vi "RT PID-DataLog - LED.vi"() -> ()   [LabVIEW 2017]
doc: "This example demonstrates how to simulate a general PID controller with alarms."
uses:
  <vilib>/Platform/TimedLoop/XDataNode/timing_clust.ctl
  <vilib>/Platform/TimedLoop/XDataNode/nitl_modes.ctl
  <vilib>/Platform/TimedLoop/XDataNode/wakeup.ctl
  <vilib>/addons/control/pid/pid.llb/PID (DBL).vi
  LogData.vi
  <vilib>/Utility/file.llb/Write Delimited Spreadsheet (DBL).vi
  <vilib>/Utility/file.llb/Write Delimited Spreadsheet (string).vi
  <vilib>/platform/TimedLoop/XDataNode/XDataNode.xnode
  <vilib>/addons/control/pid/NI_PID_pid.lvlib
  <vilib>/Platform/TimedLoop/XDataNode/XDNodeRunTimeDep.lvlib
panel:
  out "SP: Display":dbl(slide)=54.966887417218544 min=0.0 max=0.0 scale=0.0..100.0
  in  "Data Log Rate (ms)":u32=5000
  out "DataLog Loop stop":bool
  out "Data Log Loop ms":u32=5001
  out "PID Loop ms":u32=20
  in  "stop":bool
  out "Low Limit":bool
  out "High Limit":bool
  out "MV:":dbl(slide)=100.0 scale=-100.0..100.0
  out "PV:":dbl(slide)=33.01408837398299 scale=0.0..100.0
  in  "PID gains":T1={"proportional gain (Kc)"=20.0, "integral time (Ti, min)"=0.008, "derivative time (Td, min)"=0.001} {"derivative time (Td, min)" format="%.3f"; "integral time (Ti, min)" format="%.3f"; "proportional gain (Kc)" format="%.3f"}
  # "Overview: This example demonstrates how to simulate a general PID controller with alarms.\nInstructions:\n1. Run the VI and observe the Process Variable (PV) following the Setpoint (SP) value.\n2. Move the setpoint above or below the High Limit (HL) or Low Limit (LL). Verify the controls flashing when limits are reached.\n3. Change the Alarm limits to a value above or below if you are changing HL or LL, respectively and verify that the controller stop flashing.\n3. Click Stop to stop the VI."
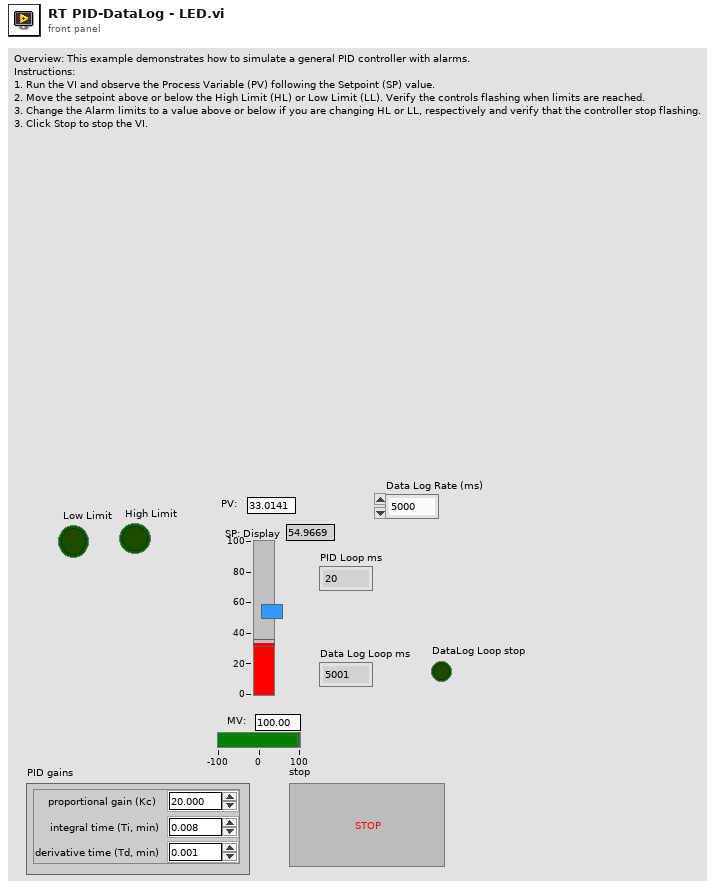
[diagram p1: front panel]
types:
  T1 = cluster{"proportional gain (Kc)":dbl, "integral time (Ti, min)":dbl, "derivative time (Td, min)":dbl}
  T2 = typedef "XDNodeRunTimeDep.lvlib/timing_clust.ctl" = cluster{"Expected End [f-1]":u64, "Actual End [f-1]":u64, "Finished Late? [f-1]":bool, "Expected End [i-1]":u64, "Actual End [i-1]":u64, "Finished Late? [i-1]":bool, "Expected Start [i]":u64, "Actual Start [i]":u64, "Expected Start [f]":u64, "Actual Start [f]":u64, "Source Name":string, "Structure Name":string, "Period":i64, "Deadline":i64, "Offset":i64, "Start":i64, "Priority":i32, "Timeout":i32, "Mode":T3, "Wakeup Reason":T4, "Error":errorcluster, "Source Type":string, "Secondary Source Type":string, "Global End Time":u64, "Global Start Time":u64, "Frame Duration":u64, "Iteration Duration":u64, "Assigned CPU":i32, "I/O Scan Engine Mode":u32}
  T3 = typedef "XDNodeRunTimeDep.lvlib/nitl_modes.ctl" = enum32{"No Change", "Process missed periods, maintain original phase", "Discard missed periods, maintain original phase", "Process missed periods, ignore original phase", "Discard missed periods, ignore original phase"}
  T4 = typedef "XDNodeRunTimeDep.lvlib/wakeup.ctl" = enum32{"Normal", "Aborted", "Asynchronous wakeup", "Timing source error", "Timed loop error", "Timeout"}
  T5 = cluster{"static gain":dbl, "lag (min)":dbl, "dead cycles":dbl, "load %":dbl, "deadband":dbl, "noise level %":dbl, "initial PV":dbl, "initial PV 2":dbl}
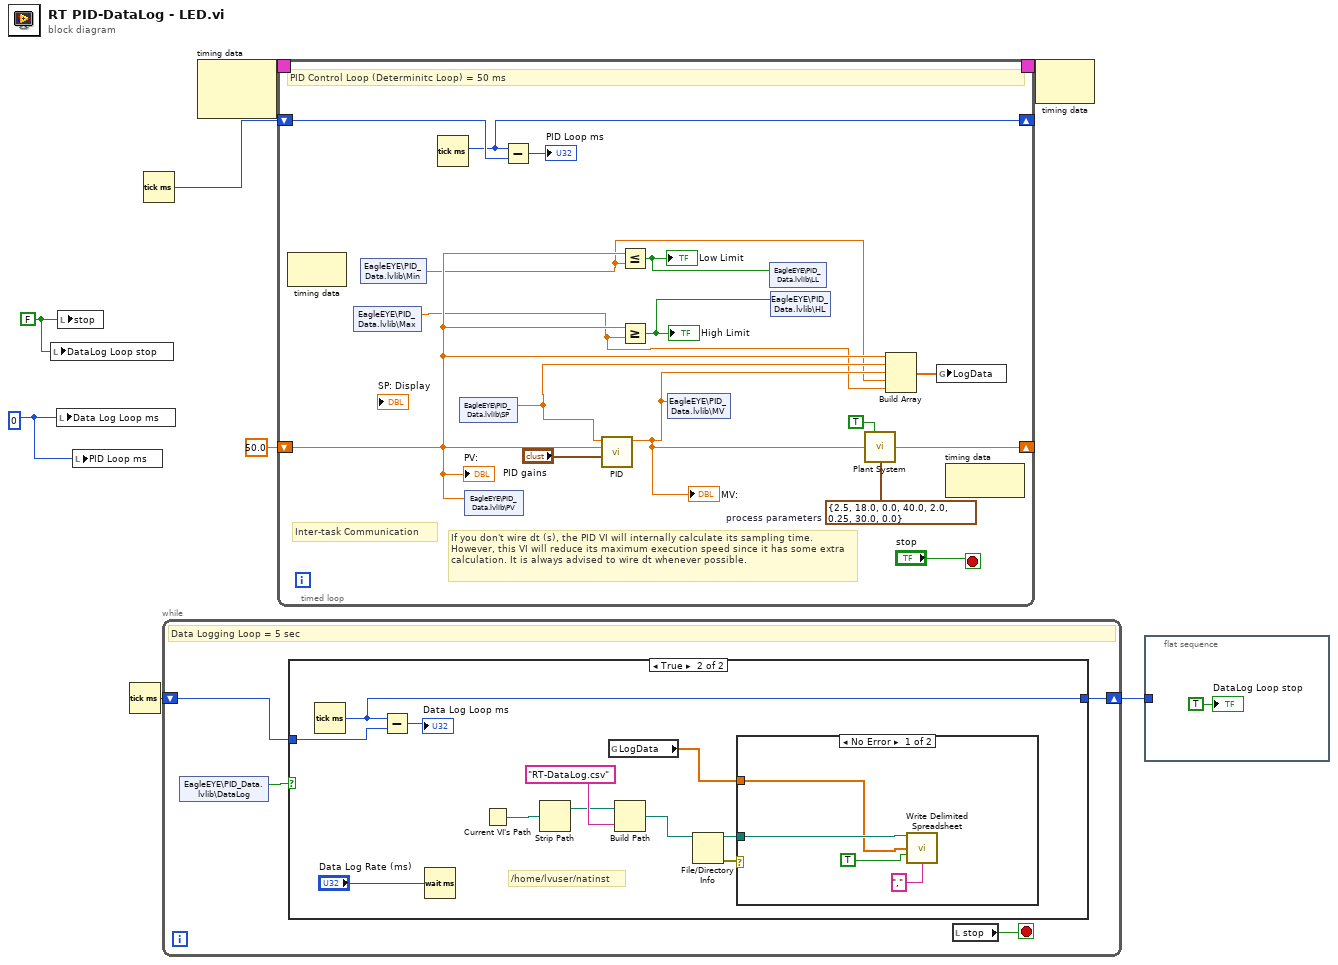
[diagram p0: block diagram]
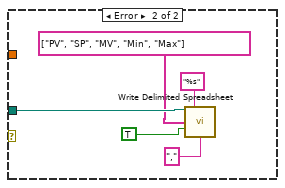
[diagram p3: hidden frame]
diagram:
  w1 = 0
  w2 = FALSE ("stop")
  n1 = local write "DataLog Loop stop"(w2) -> ()
  n2 = local write "Data Log Loop ms"(w1) -> ()
  n3 = local write "stop"(w2) -> ()
  n4 = local write "PID Loop ms"(w1) -> ()
  n5 = Tick Count (ms)() -> (millisecond timer value=w4:u32)
  n6 = Tick Count (ms)() -> (millisecond timer value=w5:u32)
  n7 = while {
    shift-right: [w10] -> w3
    shift-left: w4 -> [w11]
    stop <- w12 stop-if-true
    # "Data Logging Loop = 5 sec"
    n8 = shared-variable "EagleEYE\\PID_Data.lvlib\\DataLog"() -> (w9:bool)  [unwired: 1 in, 1 out]
    n9 = case shown="True" w9 {
      tunnel: w11 -> [w13 w15]
      tunnel: [w13 w14] -> w10
      frame False {
      }
      frame True {
        # "/home/lvuser/natinst"
        n10 = Tick Count (ms)() -> (millisecond timer value=w14:u32)
        n11 = Subtract(x=w14, y=w15) -> (x-y=→"Data Log Loop ms":u32)
        n12 = Wait (ms)(milliseconds to wait="Data Log Rate (ms)") -> ()  [unwired: 1 out]
        n13 = Current VI's Path() -> (path=w22:path)
        n14 = Strip Path(path=w22) -> (stripped path=w20:path)  [unwired: 1 out]
        n15 = global read "LogData.vi" "LogData"() -> (w23:dbl[])
        n16 = Build Path(base path=w20, name or relative path="RT-DataLog.csv") -> (appended path=w19:path)
        n17 = File/Directory Info(path=w19) -> (path out=w17:path, error out=w18:errorcluster)  [unwired: 1 in, 5 out]
        n18 = case shown="No Error" w18 {
          tunnel: w23 -> [w25 _]
          tunnel: w17 -> [w28 w33]
          frame No Error {
            n19 = call-poly <vilib>:"Write Delimited Spreadsheet.vi"("file path (dialog if empty)"=w28, "1D data"=w25, "append to file? (new file:F)"=TRUE, "delimiter (\\t)"="," ("delimiter (\\t)")) -> ()  [unwired: 10 in, 2 out]
          }
          frame Error {
            n20 = call-poly <vilib>:"Write Delimited Spreadsheet.vi"("file path (dialog if empty)"=w33, "format (%s)"="%s", "1D data"=string[] ["PV", "SP", "MV", "Min", "Max"], "append to file? (new file:F)"=TRUE, "delimiter (\\t)"="," ("delimiter (\\t)")) -> ()  [unwired: 9 in, 2 out]
          }
        }
      }
    }
    n21 = local read "stop"() -> (w12:bool)
  }
  n22 = node-c288() -> (w7:T2)  [unwired: 2 in]
  n23 = timed-loop {
    shift-left: 50.0 ("Plant Output") -> [w38]
    shift-right: [w49] -> _
    timing: w7 -> [_]
    timing-out: [_] -> w6
    shift-right: [w43] -> _
    shift-left: w5 -> [w44]
    stop <- "stop" stop-if-true
    w47 = T5 {"static gain"=2.5, "lag (min)"=18.0, "dead cycles"=0.0, "load %"=40.0, "deadband"=2.0, "noise level %"=0.25, "initial PV"=30.0, "initial PV 2"=0.0}  # process parameters
    # "Inter-task Communication"
    # "If you don't wire dt (s), the PID VI will internally calculate its sampling time. However, this VI will reduce its maximum execution speed since it has some extra calculation. It is always advised to wire dt whenever possible."
    # "PID Control Loop (Determinitc Loop) = 50 ms"
    n24 = node-c288() -> ()  [unwired: 1 in, 1 out]
    n25 = shared-variable "EagleEYE\\PID_Data.lvlib\\Max"() -> (w34:dbl)  [unwired: 1 in, 1 out]
    n26 = shared-variable "EagleEYE\\PID_Data.lvlib\\Min"() -> (w35:dbl)  [unwired: 1 in, 1 out]
    n27 = Tick Count (ms)() -> (millisecond timer value=w43:u32)
    n28 = shared-variable "EagleEYE\\PID_Data.lvlib\\SP"() -> (w37:dbl)  [unwired: 1 in, 1 out]
    n29 = shared-variable "EagleEYE\\PID_Data.lvlib\\PV"(w38) -> ()  [unwired: 1 in, 1 out]
    n30 = Subtract(x=w43, y=w44) -> (x-y=→"PID Loop ms":u32)
    n31 = call-poly <vilib>:"PID.vi"("PID gains"="PID gains", "process variable"=w38, "setpoint"=w37) -> ("output"=w36:dbl)  [unwired: 7 in, 1 out]
    "MV:" <- w36
    n32 = Less Or Equal?(x=w38, y=w35) -> (x <= y?=w41:bool)
    "Low Limit" <- w41
    n33 = Greater Or Equal?(x=w38, y=w34) -> (x >= y?=w40:bool)
    "High Limit" <- w40
    n34 = shared-variable "EagleEYE\\PID_Data.lvlib\\MV"(w36) -> ()  [unwired: 1 in, 1 out]
    n35 = shared-variable "EagleEYE\\PID_Data.lvlib\\LL"(w41) -> ()  [unwired: 1 in, 1 out]
    n36 = shared-variable "EagleEYE\\PID_Data.lvlib\\HL"(w40) -> ()  [unwired: 1 in, 1 out]
    n37 = call "Plant System.vi"("Integrator ?"=TRUE, "Plant Input"=w36, "process parameters"=w47) -> ("Plant Output"=w49:dbl)  [unwired: 12 in]
    n38 = Build Array(w38, w37, w36, w35, w34) -> (w39:dbl[])
    n39 = global write "LogData.vi" "LogData"(w39) -> ()
    n40 = node-c288() -> ()  [unwired: 1 in, 1 out]
    "PV:" <- w38
  }
  n41 = node-c288(w6) -> ()  [unwired: 1 out]
  n42 = flat-sequence {
    tunnel: w3 -> [_]
    frame #0 {
      "DataLog Loop stop" <- TRUE ("DataLog Loop stop")
    }
  }
